vi "divide.vi"(8 "error in (no error)":errorcluster, 10 "b":i32, 11 "a":i32) -> (0 "error out":errorcluster, 3 "function return":sgl format="%#.2f")   [LabVIEW 2021, in "new_libmath.lvlib"]
doc: "float divide(int a, int b);"
uses:
  <userlib>/new_libmath/new_libmath.lvlib
  <userlib>/new_libmath/libmath.dll
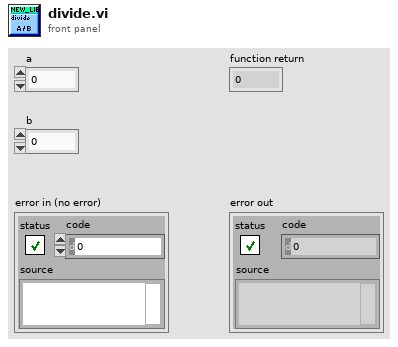
[diagram p1: front panel]
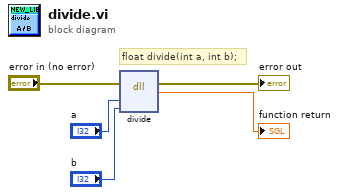
[diagram p0: block diagram]
diagram:
  # "float divide(int a, int b);"
  n1 = dll-call lib="C:/Program Files (x86)/National Instruments/LabVIEW 2021/user.lib/new_libmath/libmath.*" fn="divide"(error in="error in (no error)", "a"="a", "b"="b") -> (error out=→"error out":errorcluster, "return type"=→"function return":sgl)  [unwired: 4 in, 1 out]
